vi "Initialize Shared Variables Host.vi"(8 "error in (no error)":errorcluster, 11 "IP Address (No Slashes)":string) -> (0 "error out":errorcluster, 3 "Shared Variable References":T1)   [LabVIEW 2015]
doc: "This VI takes an IP address and builds references to all the shared variables used on the host."
uses:
  Custom Controls/Display State.ctl
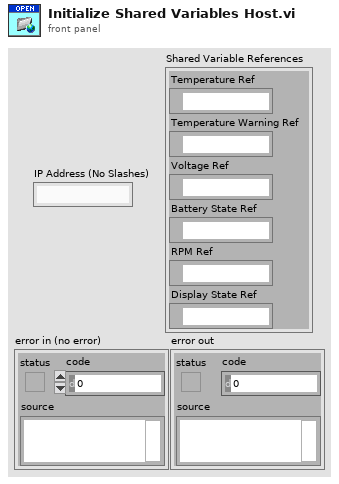
[diagram p1: front panel]
types:
  T1 = cluster{"Temperature Ref":refnum<k21>, "Temperature Warning Ref":refnum<k21>, "Voltage Ref":refnum<k21>, "Battery State Ref":refnum<k21>, "RPM Ref":refnum<k21>, "Display State Ref":refnum<k21>}
  T2 = typedef "Display State.ctl" = enum16{"Battery State", "RPM", "Temp", "Voltage"}
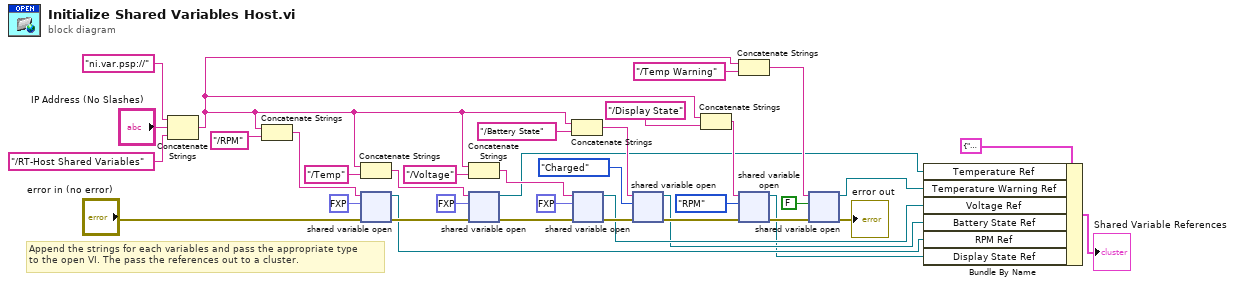
[diagram p0: block diagram]
diagram:
  # "Append the strings for each variables and pass the appropriate type\nto the open VI. The pass the references out to a cluster."
  n1 = Concatenate Strings("ni.var.psp://", "IP Address (No Slashes)", "/RT-Host Shared Variables") -> (w1:string)
  n2 = Concatenate Strings(w1, "/RPM") -> (w30:string)
  n3 = Concatenate Strings(w1, "/Temp") -> (w34:string)
  n4 = shared-variable-open(w30, "error in (no error)", fxp<+,32,16> 0.0 ("RPM")) -> (w8:refnum<k21>, w24:errorcluster)  [unwired: 1 in]
  n5 = Concatenate Strings(w1, "/Voltage") -> (w33:string)
  n6 = shared-variable-open(w34, w24, fxp<+/-,32,13> 0.0 ("Temp")) -> (w12:refnum<k21>, w23:errorcluster)  [unwired: 1 in]
  n7 = Concatenate Strings(w1, "/Battery State") -> (w26:string)
  n8 = shared-variable-open(w33, w23, fxp<+/-,24,5> 0.0 ("Voltage")) -> (w10:refnum<k21>, w22:errorcluster)  [unwired: 1 in]
  n9 = shared-variable-open(w26, w22, enum16{"Charged", "Running", "Low Batt"}."Charged" ("Battery State")) -> (w9:refnum<k21>, w21:errorcluster)  [unwired: 1 in]
  n10 = Concatenate Strings(w1, "/Display State") -> (w28:string)
  n11 = Concatenate Strings(w1, "/Temp Warning") -> (w31:string)
  n12 = shared-variable-open(w28, w21, Display_State."RPM" ("Display State")) -> (w7:refnum<k21>, w20:errorcluster)  [unwired: 1 in]
  n13 = shared-variable-open(w31, w20, FALSE ("Temp Warning")) -> (w11:refnum<k21>, →"error out":errorcluster)  [unwired: 1 in]
  n14 = Bundle By Name(cluster=T1 {"Temperature Ref"="", "Temperature Warning Ref"="", "Voltage Ref"="", "Battery State Ref"="", "RPM Ref"="", "Display State Ref"=""}, "Temperature Ref"=w12, "Temperature Warning Ref"=w11, "Voltage Ref"=w10, "Battery State Ref"=w9, "RPM Ref"=w8, "Display State Ref"=w7) -> (→"Shared Variable References":T1)
